vi "Send scan_perform_scan.vi"(7 "Message Priority (Normal)":T4=enum."Normal", 8 "error in (no error)":errorcluster, 10 "scan_settings":T1={"Center Pos. (mm)"=0.0, "Range [--|--]"=0.0, "Unit"=enum."mm", "Steps"=0.0, "Stage Number"=enum."1", "Stage Speed"=1.0, "Dwell Time (s)"=0.1, "Record Type"=enum."hdf5", "Save Path"=path "", "Notes"=""}, 11 "Message Enqueuer":refnum<class "Message Enqueuer.lvclass">) -> (0 "error out":errorcluster, 3 "Message Enqueuer out":refnum<class "Message Enqueuer.lvclass">)   [LabVIEW 2015, in "scan_perform_scan Msg.lvclass"]
doc: "This VI sends the message to an actor."
uses:
  scan_perform_scan Msg.lvclass
  <vilib>/ActorFramework/Message Enqueuer/Message Enqueuer.lvclass
  <vilib>/ActorFramework/Message Enqueuer/Message Priority.ctl
  Scan/scan_settings.ctl
  Scan/scan_unit.ctl
  Scan/scan_record.ctl
  scan_perform_scan Msg.lvclass/scan_perform_scan Msg.ctl
  <vilib>/ActorFramework/Message Enqueuer/Message Enqueuer.lvclass/Message Enqueuer.ctl
  <vilib>/ActorFramework/Message Priority Queue/Priority Enqueue.vi
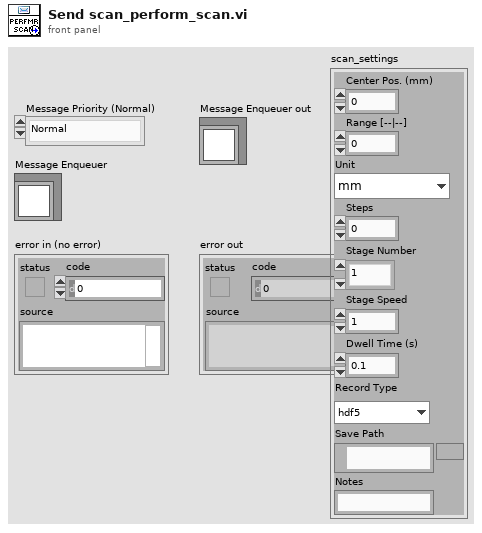
[diagram p1: front panel]
types:
  T1 = typedef "scan_settings.ctl" = cluster{"Center Pos. (mm)":dbl, "Range [--|--]":dbl, "Unit":T2, "Steps":dbl, "Stage Number":enum16{"1", "2"}, "Stage Speed":dbl, "Dwell Time (s)":dbl, "Record Type":T3, "Save Path":path, "Notes":string}
  T2 = typedef "scan_unit.ctl" = enum16{"mm", "s", "ms", "us", "ns", "ps", "fs"}
  T3 = typedef "scan_record.ctl" = enum16{"hdf5", "legacy", "None"}
  T4 = typedef "Actor Framework.lvlib/Message Enqueuer.lvclass/Message Priority.ctl" = enum16{"Low", "Normal", "High"}
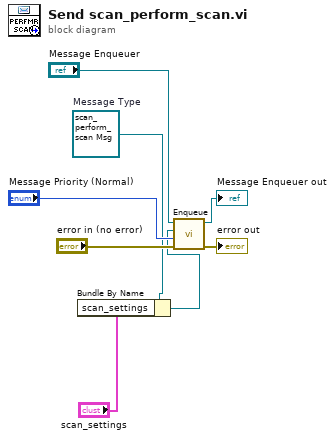
[diagram p0: block diagram]
diagram:
  w3 = refnum<class "scan_perform_scan Msg.lvclass"> refnum  # Message Type
  n1 = Bundle By Name(cluster=w3, "scan_settings"="scan_settings") -> (w2:refnum<class "scan_perform_scan Msg.lvclass">)
  n2 = call <vilib>:"Enqueue.vi"("error in (no error)"="error in (no error)", "Message Priority (Normal)"="Message Priority (Normal)", "Message"=w2, "Message Enqueuer in"="Message Enqueuer") -> ("error out"=→"error out":errorcluster, "Message Enqueuer out"=→"Message Enqueuer out":refnum<class "Message Enqueuer.lvclass">)  [unwired: 6 in]
